vi "2-DSpecView.vi"() -> ()   [LabVIEW 2022 SP3]
uses:
  <vilib>/Utility/file.llb/Read From Spreadsheet File (DBL).vi
panel:
  in  "Zero Pad?":bool
  in  "Log scaling?":bool=TRUE
  in  "Cal File Selection":u16(ring) items=["Don't subtract a Cal File", "Use Info in Header", "Specify Cal Info"]
  out "need this ROI to\nmatch Cal File":i32
  in  "RF File Att":dbl format="%.2f"
  in  "Cal File Att":dbl format="%.2f"
  in  "Cal File Name":string
  out "2 D FFT (x scale in MHz, magnitude in dB)":dbl[][](graph)
  out "raw x coord":dbl[][](array[numeric]) format="%.2f"
  out "raw y coord":dbl[][](array[numeric]) format="%.2f"
  out "raw sector image":dbl[][](array[numeric]) format="%.2f"
  out "Axis scaling Params":T1 {"Y high" format="%.2f"; "Y low" format="%.2f"; "X left" format="%.2f"; "X right" format="%.2f"}
  out "Sector as data array":dbl[][](graph)
  in  "Last sector file":path
  in  "View Header?":bool
  in  "FFT size for":u16(ring)=6 items=["next 2^n", "8", "16", "32", "64", "128", "256", "512"]
  out "Raw data":i16[][](graph)
  in  "new eye file path":path
  # "Select region to provide 3-D manipulation.\nKeep RED curser above and to left of blue."
  # "Blue curser controls upper right of sector ROI,\nRed curser controls lower left."
  # "© 2000 Riverside Research Institute"
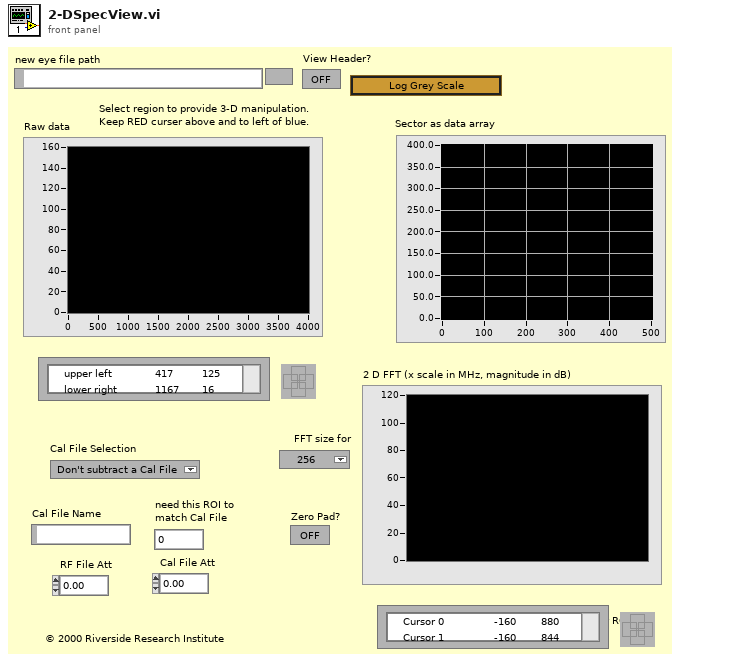
[diagram p1: front panel]
types:
  T1 = cluster{"X right":dbl, "X left":dbl, "Y low":dbl, "Y high":dbl}
  T2 = cluster{"# rf points per line":u16, "# lines per scan":u16, "sample rate MHz":u16, "# A/D bits":u16, "# bytes per A/D":u16, "TGC Flag":u16, "A/D Type":string}
  T3 = cluster{"delay":sgl, "pivot distance":sgl, "sector scan angle":sgl, "operator":string, "Scan Mode":string, "location":string}
  T4 = cluster{"RF file name":string, "RF file att":string, "RF cal file name":string, "RF cal file att":string}
  T5 = cluster{"Cursor.Cursor X":dbl, dbl, "Cursor.Cursor Y":dbl, dbl}
  T6 = cluster{"Cursor.Cursor X":i32, i32, "Cursor.Cursor Y":i32, i32}
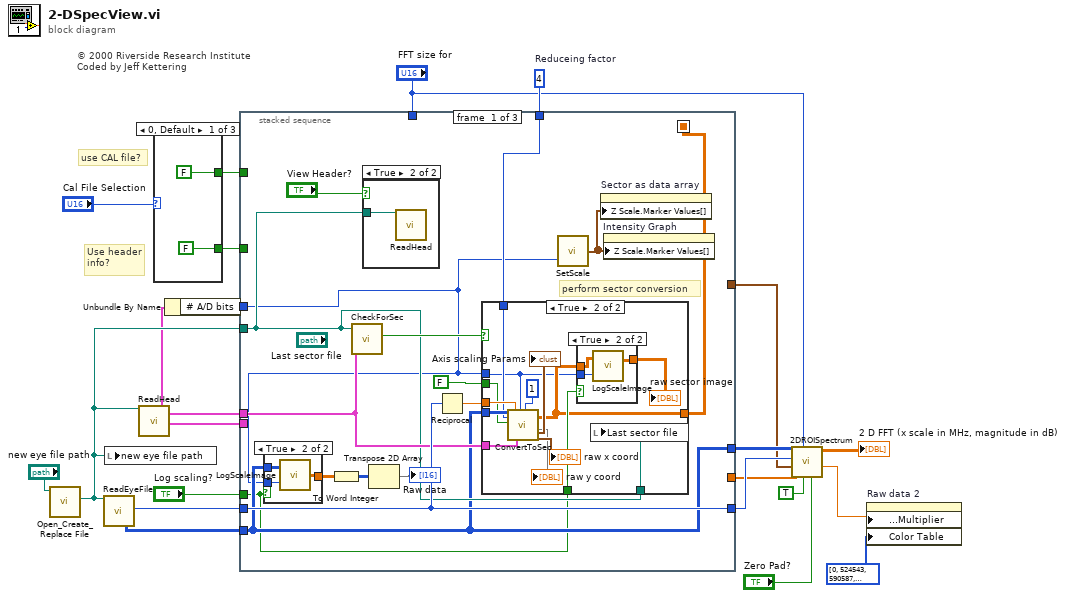
[diagram p0: block diagram]
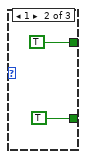
[diagram p2: hidden frame]
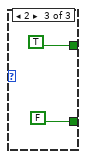
[diagram p3: hidden frame]
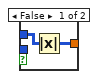
[diagram p4: hidden frame]
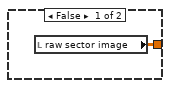
[diagram p6: hidden frame]
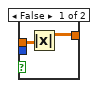
[diagram p7: hidden frame]
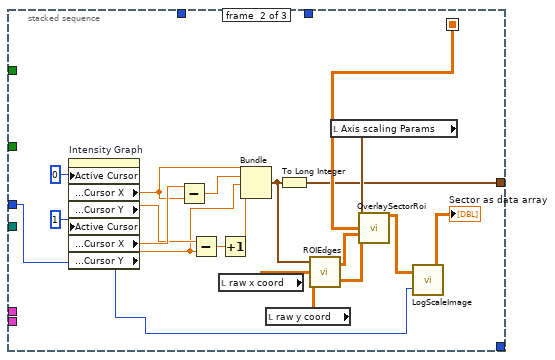
[diagram p8: hidden frame]
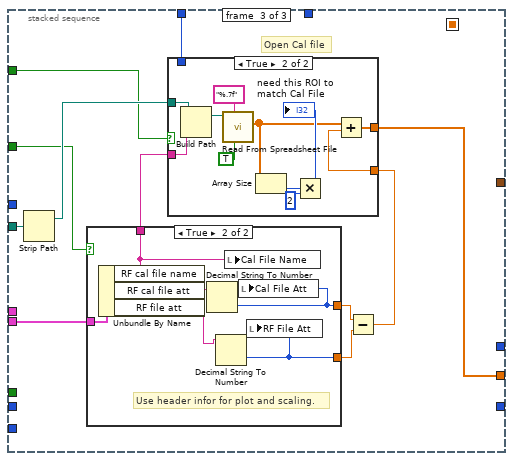
[diagram p9: hidden frame]
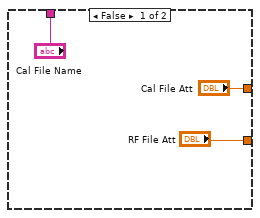
[diagram p10: hidden frame]
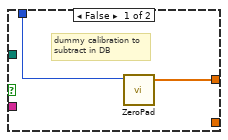
[diagram p11: hidden frame]
diagram:
  w19 = 4  # Reduceing factor
  # "© 2000 Riverside Research Institute\nCoded by Jeff Kettering"
  # "use CAL file?"
  # "Use header\ninfo?"
  n1 = call <vilib>:"Open_Create_Replace File.vi"("file path"="new eye file path") -> ("new file path"=w20:path)  [unwired: 5 in, 5 out]
  n2 = call "ReadEyeFile.vi"("new file path"=w20) -> ("2-D data array"=w3:i16[][], "sample rate MHz"=w22:u16)  [unwired: 1 in, 16 out]
  n3 = local write "new eye file path"(w20) -> ()
  n4 = call "ReadHead.vi"("new file path"=w20) -> ("A/D info"=w2:T2, "Scan Info"=w21:T3, "RF Info"=w11:T4)  [unwired: 16 out]
  n5 = case shown="0, Default" "Cal File Selection" {
    tunnel: [FALSE TRUE TRUE] -> w9
    tunnel: [FALSE TRUE FALSE] -> w8
    frame 0, Default {
    }
    frame 1 {
    }
    frame 2 {
    }
  }
  n6 = Unbundle By Name(w2) -> ("# A/D bits"=w1:u16)
  n7 = stacked-sequence {
    seq-local: [w42 _ _] -> [_ w91 _]
    tunnel: w22 -> [w44 _ _]
    tunnel: w3 -> [w35 _ _]
    tunnel: w21 -> [w39 _ _]
    tunnel: [_ w81 _] -> w16
    tunnel: [w44 _ _] -> w17
    tunnel: [w35 _ _] -> w18
    tunnel: w20 -> [w38 _ w100]
    tunnel: w19 -> [w41 _ _]
    tunnel: w11 -> [_ _ w99]
    tunnel: w9 -> [_ _ w98]
    tunnel: w8 -> [_ _ w97]
    tunnel: "FFT size for" -> [_ _ w96]
    tunnel: [_ _ w95] -> w6
    tunnel: "Log scaling?" -> [w34 _ _]
    tunnel: w1 -> [w30 w72 _]
    frame #0 {
      # "perform sector conversion"
      n8 = case shown="True" w34 {
        tunnel: [w46 w49] -> w36
        tunnel: w35 -> [w47 w50]
        tunnel: w30 -> [_ w48]
        frame False {
          n9 = Absolute Value(x=w47) -> (abs(x)=w46:i16[][])
        }
        frame True {
          n10 = call "LogScaleImage.vi"("A/D bits"=w48, "input array"=w50) -> ("log scale image"=w49:dbl[][])  [unwired: 1 out]
        }
      }
      n11 = To Word Integer(number=w36) -> (16bit integer=w37:i16[][])
      n12 = call "CheckForSec.vi"("Scan Info"=w39, "Current file"=w38) -> ("sector?"=w40:bool)  [unwired: 1 in, 6 out]
      n13 = case shown="True" "View Header?" {
        tunnel: w38 -> [_ w51]
        frame False {
        }
        frame True {
          n14 = call "ReadHead.vi"("new file path"=w51) -> ()  [unwired: 19 out]
        }
      }
      n15 = Transpose 2D Array(2D array=w37) -> (transposed array=→"Raw data":i16[][])
      n16 = Reciprocal(x=w44) -> (1/x=w45:dbl)
      n17 = case shown="True" w40 {
        tunnel: [w52 w57] -> w42
        tunnel: w35 -> [_ w66]
        tunnel: w39 -> [_ w65]
        tunnel: w45 -> [_ w64]
        tunnel: w38 -> [_ w63]
        tunnel: w41 -> [_ w59]
        tunnel: w34 -> [_ w58]
        tunnel: w30 -> [_ w55]
        tunnel: FALSE ("no oversample?") -> [_ w53]
        frame False {
          n18 = local read "raw sector image"() -> (w52:dbl[][])
        }
        frame True {
          n19 = call "ConvertToSec.vi"("raw image data in"=w66, "reduce pts by factor of"=w59, "Add Lines"=w53, "Time between rf pts\nmicros"=w64, "Scan Info"=w65, "Abs?"=w55, "Smooth factor"=1) -> (13:→"raw y coord", "raw sector out"=w57:dbl[][], "Axis scaling Params"=→"Axis scaling Params":T1, "scales"=→"raw x coord":cluster{"inc x (mm)":dbl, "inc y (mm)":dbl})  [unwired: 4 in, 5 out]
          n20 = case shown="True" w58 {
            tunnel: [w67 w71] -> w56
            tunnel: w57 -> [w68 w70]
            tunnel: w55 -> [_ w69]
            frame False {
              n21 = Absolute Value(x=w68) -> (abs(x)=w67:dbl[][])
            }
            frame True {
              n22 = call "LogScaleImage.vi"("A/D bits"=w69, "input array"=w70) -> ("log scale image"=w71:dbl[][])  [unwired: 1 out]
            }
          }
          "raw sector image" <- w56
          n23 = local write "Last sector file"(w63) -> ()
        }
      }
      n24 = call "SetScale.vi"("# A/D bits"=w30) -> ("Array"=w33:cluster{dbl, u32}[])  [unwired: 1 in]
      n25 = property on="Sector as data array" class="IntGraph (strict)"("Z Scale.Marker Values[]"=w33) -> ()  [unwired: 2 in, 2 out]
      n26 = property on="Intensity Graph" class="IntGraph (strict)"("Z Scale.Marker Values[]"=w33) -> ()  [unwired: 2 in, 2 out]
    }
    frame #1 {
      n27 = property on="Intensity Graph" class="IntGraph (strict)"("Active Cursor"=u32 0 ("Write Attribute"), "Active Cursor"=u32 1 ("Write Attribute")) -> ("Cursor.Cursor Position:Cursor X"=w86:dbl, "Cursor.Cursor Position:Cursor Y"=w89:dbl, "Cursor.Cursor Position:Cursor X"=w90:dbl, "Cursor.Cursor Position:Cursor Y"=w84:dbl)  [unwired: 2 in, 2 out]
      n28 = Subtract(x=w90, y=w86) -> (x-y=w85:dbl)
      n29 = Subtract(x=w89, y=w84) -> (x-y=w83:dbl)
      n30 = local read "raw x coord"() -> (w79:dbl[][])
      n31 = Increment(x=w83) -> (x+1=w75:dbl)
      n32 = Bundle("Cursor.Cursor X"=w86, w85, "Cursor.Cursor Y"=w84, w75) -> (w78:T5)  [unwired: 1 out]
      n33 = local read "raw y coord"() -> (w80:dbl[][])
      n34 = To Long Integer(number=w78) -> (32bit integer=w81:T6)
      n35 = call "ROIEdges.vi"("Array Subset"=w78, "raw x coord"=w79, "raw y coord"=w80) -> ("x box"=w77:dbl[][], "y box"=w76:dbl[][])  [unwired: 2 in]
      n36 = local read "Axis scaling Params"() -> (w82:T1)
      n37 = call "OverlaySectorRoi.vi"("Axis scaling Params"=w82, "Sector as Array"=w91, "x coord"=w77, "y coord"=w76) -> ("image overlay"=w74:dbl[][])  [unwired: 3 in, 8 out]
      n38 = call "LogScaleImage.vi"("A/D bits"=w72, "input array"=w74) -> ("log scale image"=→"Sector as data array":dbl[][])  [unwired: 1 out]
    }
    frame #2 {
      # "Open Cal file"
      n39 = Strip Path(path=w100) -> (stripped path=w101:path)  [unwired: 1 out]
      n40 = case shown="True" w97 {
        tunnel: ["Cal File Att" w109] -> w94
        tunnel: ["RF File Att" w108] -> w93
        tunnel: ["Cal File Name" w107] -> w102
        tunnel: w99 -> [_ w106]
        frame False {
          # "use input data for fit and plot scaling"
        }
        frame True {
          # "Use header infor for plot and scaling."
          n41 = Unbundle By Name(w106) -> ("RF cal file name"=w107:string, "RF cal file att"=w111:string, "RF file att"=w110:string)
          n42 = Decimal String To Number(string=w111) -> (number=w109:i32)  [unwired: 3 out]
          n43 = Decimal String To Number(string=w110) -> (number=w108:i32)  [unwired: 3 out]
          n44 = local write "Cal File Name"(w107) -> ()
          n45 = local write "Cal File Att"(w109) -> ()
          n46 = local write "RF File Att"(w108) -> ()
        }
      }
      n47 = Subtract(x=w94, y=w93) -> (x-y=w92:dbl)
      n48 = case shown="True" w98 {
        tunnel: w102 -> [_ w124]
        tunnel: w101 -> [_ w117]
        tunnel: [w112 w114] -> w95
        tunnel: w96 -> [w113 _]
        tunnel: w92 -> [_ w116]
        frame False {
          # "dummy calibration to\nsubtract in DB"
          n49 = call "ZeroPad.vi"("FFT size"=w113) -> ("Ouput Array"=w112:dbl[])  [unwired: 1 in, 4 out]
        }
        frame True {
          n50 = Build Path(base path=w117, name or relative path=w124) -> (appended path=w123:path)
          n51 = call-poly <vilib>:"Read From Spreadsheet File.vi"("transpose (no:F)"=TRUE, "format (%.3f)"="%.7f", "file path (dialog if empty)"=w123) -> ("first row"=w115:dbl[])  [unwired: 1 in, 7 out]
          n52 = Array Size(array=w115) -> (size(s)=w121:i32)
          n53 = Multiply(x=w121, y=2) -> (x*y=→"need this ROI to\nmatch Cal File":i32)
          n54 = Add(x=w115, y=w116) -> (x+y=w114:dbl[])
        }
      }
    }
  }
  n55 = call "2DROISpectrum.vi"("Zero Pad?"="Zero Pad?", "convert output to dB?"=TRUE, "FFT size"="FFT size for", "Cal File"=w6, "Array Subset"=w16, "freq (MHz)"=w17, "2-D data array"=w18) -> ("df (MHz)"=w12:dbl, "power spectrum in dB"=→"2 D FFT (x scale in MHz, magnitude in dB)":dbl[][])  [unwired: 3 out]
  n56 = property on="Raw data 2" class="IntGraph (strict)"("X Scale.Offset and Multiplier:Multiplier"=w12, "Color Table"=u32[] [0, 524543, 590587, 591095, 657139, 657647, 723691, 724455, 790500, 791008, 857052, 923096, 923604, 989648, 990156, 1056200, 1056708, 1122752, 1123516, 1189560, 1255604, 1256113, 1322157, 1322665, 1388709, 1389217, 1455261, 1521305, 1521816, 1588120, 1588631, 1654678, 1655190, 1721237, 1721748, 1787796, 1853843, 1854354, 1920402, 1920913, 1987216, 1987728, 2053775, 2054286, 2120334, 2186381, 2186892, 2252940, 2253451, 2319498, 2320009, 2386313, 2386824, 2452871, 2518919, 2519430, 2585477, 2585989, 2652036, 2652547, 2718595, 2719106, 2785409, 2851457, 2851968, 2918015, 2918527, 2984574, 2985085, 3051133, 3051644, 3117691, 3183739, 3184250, 3250553, 3251065, 3317112, 3317623, 3383671, 3449718, 3450229, 3516277, 3516788, 3582835, 3583347, 3649650, 3650161, 3716209, 3782256, 3782767, 3848815, 3849326, 3915373, 3915885, 3981932, 3982443, 4048746, 4114794, 4115305, 4181352, 4181864, 4247911, 4248422, 4314470, 4314981, 4381028, 4447076, 4447843, 4513890, 4514402, 4580449, 4580960, 4647008, 4647519, 4713566, 4779614, 4780125, 4846172, 4846940, 4912987, 4913498, 4979546, 5045593, 5046104, 5111128, 5110615, 5175638, 5175126, 5240149, 5239636, 5304660, 5369683, 5369170, 5434450, 5433937, 5498960, 5498448, 5563471, 5562958, 5627982, 5693005, 5823564, 5888587, 6019147, 6084170, 6214729, 6279753, 6410312, 6475335, 6605895, 6670918, 6801477, 6866757, 6997316, 7062339, 7192899, 7257922, 7388481, 7453505, 7584064, 7649087, 7779647, 7844670, 7909693, 8040253, 8105276, 8235835, 8300859, 8431418, 8496441, 8627257, 8692280, 8822839, 8887863, 9018422, 9083445, 9214005, 9279028, 9409587, 9474611, 9605170, 9670193, 9800753, 9865776, 9996335, 10061359, 10126382, 10256941, 10321964, 10452780, 10517803, 10648362, 10713386, 10843945, 10908968, 11039528, 11104551, 11235110, 11300134, 11430693, 11495716, 11626276, 11691299, 11821858, 11886882, 12017441, 12082464, 12213024, 12278303, 12343326, 12473886, 12538909, 12669468, 12734492, 12865051, 12930074, 13060634, 13125657, 13256216, 13321240, 13451799, 13516822, 13647382, 13712405, 13842964, 13907988, 14038803, 14103826, 14234386, 14299409, 14429968, 14494992, 14560015, 14690574, 14755597, 14886157, 14951180, 15081739, 15146763, 15277322, 15342345, 15472905, 15537928, 15668487, 15733511, 15864326, 15929349, 16059909, 16124932, 16255491, 16320515, 16451074, 16516097, 16646657, 16711680, 16711680]) -> ()  [unwired: 2 in, 2 out]
